vi "ScanString.vi"(8 "error in (no error)":errorcluster, 10 "String":string, 11 "Bool D Element in":refnum<class "Bool D Element.lvclass">) -> (0 "error out":errorcluster, 3 "Bool D Element out":refnum<class "Bool D Element.lvclass">)   [LabVIEW 2020, in "D Datagrid Library.lvlib" / "Bool D Element.lvclass"]
uses:
  Bool D Element.lvclass
  Bool D Element.lvclass/Bool D Element.ctl
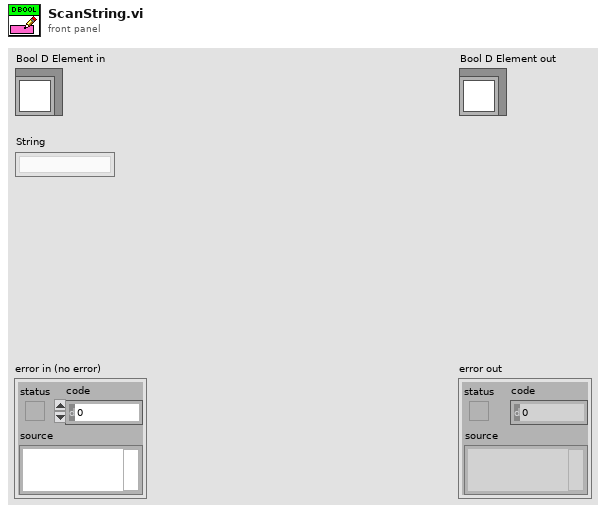
[diagram p1: front panel]
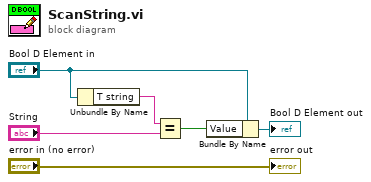
[diagram p0: block diagram]
diagram:
  n1 = Unbundle By Name("Bool D Element in") -> ("T string"=w6:string)
  n2 = Equal?(x=w6, y="String") -> (x = y?=w1:bool)
  n3 = Bundle By Name(cluster="Bool D Element in", "Value"=w1) -> (→"Bool D Element out":refnum<class "Bool D Element.lvclass">)
  "error out" <- "error in (no error)"
